vi "CalcSliderProgress.vi"(9 "Next Position":dbl, 10 "Array":T1(array[cluster]) {"Start" format="%<%.3X>T"}, 11 "Time Stamp":timestamp) -> (3 "Slider Progress":dbl)   [LabVIEW 2017]
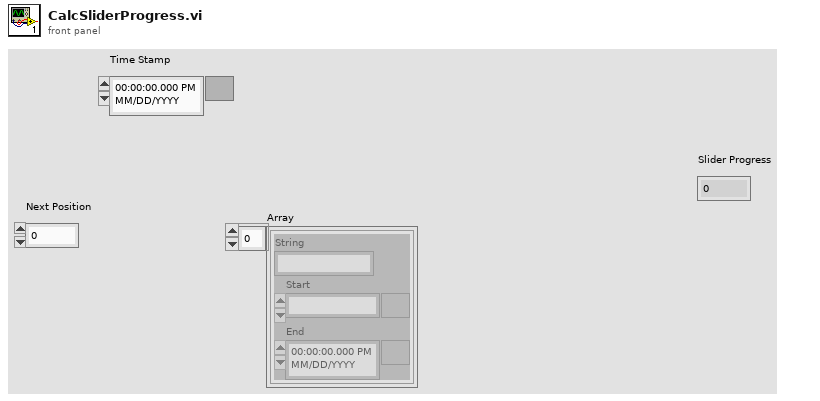
[diagram p1: front panel]
types:
  T1 = cluster{"String":string, "Start":timestamp, "End":timestamp}[]
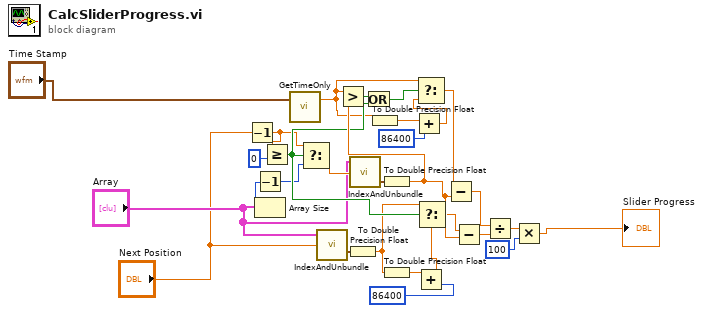
[diagram p0: block diagram]
diagram:
  n1 = Decrement(x="Next Position") -> (x-1=w20:dbl)
  n2 = Array Size(array="Array") -> (size(s)=w18:i32)
  n3 = Decrement(x=w18) -> (x-1=w19:i32)
  n4 = Greater Or Equal?(x=w20, y=0) -> (x >= y?=w25:bool)
  n5 = call "GetTimeOnly.vi"("Time Stamp"="Time Stamp") -> ("Numeric"=w4:dbl)  [unwired: 2 in]
  n6 = Select(t=w20, s=w25, f=w19) -> (s? t:f=w28:dbl)
  n7 = call "IndexAndUnbundle.vi"("Index"="Next Position", "Array"="Array") -> ("Start"=w26:timestamp)  [unwired: 1 in, 2 out]
  n8 = To Double Precision Float(number=w26) -> (double precision float=w8:dbl)
  n9 = call "IndexAndUnbundle.vi"("Index"=w28, "Array"="Array") -> ("End"=w27:timestamp)  [unwired: 1 in, 2 out]
  n10 = To Double Precision Float(number=w4) -> (double precision float=w2:dbl)
  n11 = To Double Precision Float(number=w27) -> (double precision float=w29:dbl)
  n12 = Greater?(x=w4, y=w29) -> (0:w23:bool)
  n13 = Or(x=w23, y=w25) -> (x .or. y?=w24:bool)
  n14 = To Double Precision Float(number=w8) -> (double precision float=w7:dbl)
  n15 = Add(x=w2, y=86400) -> (x+y=w1:dbl)
  n16 = Select(t=w4, s=w24, f=w1) -> (s? t:f=w22:dbl)
  n17 = Add(x=w7, y=86400) -> (x+y=w5:dbl)
  n18 = Select(t=w8, s=w25, f=w5) -> (s? t:f=w21:dbl)
  n19 = Subtract(x=w22, y=w29) -> (x-y=w13:dbl)
  n20 = Subtract(x=w21, y=w29) -> (x-y=w14:dbl)
  n21 = Divide(x=w13, y=w14) -> (x/y=w16:dbl)
  n22 = Multiply(x=w16, y=100) -> (x*y=→"Slider Progress":dbl)
